vi "Data processing_average_injection (SubVI).vi"(0 "Measurement input":string) -> (20 "output cluster 2":T1, 27 "output cluster":cluster{bool, bool, bool, bool, bool, bool})   [LabVIEW 2014]
uses:
  <vilib>/Analysis/NI_AALBase.lvlib
  <vilib>/Analysis/baseanly.llb/Mean (DBL).vi
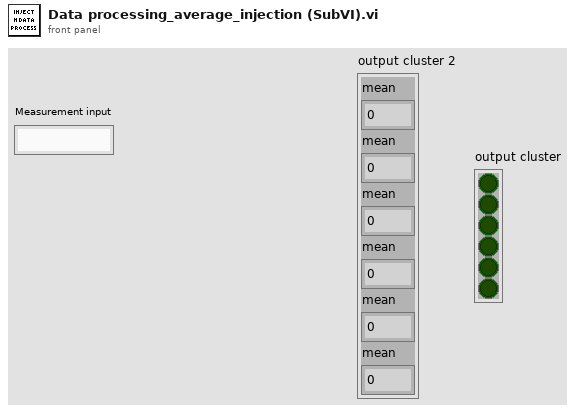
[diagram p1: front panel]
types:
  T1 = cluster{"mean":dbl, "mean":dbl, "mean":dbl, "mean":dbl, "mean":dbl, "mean":dbl}
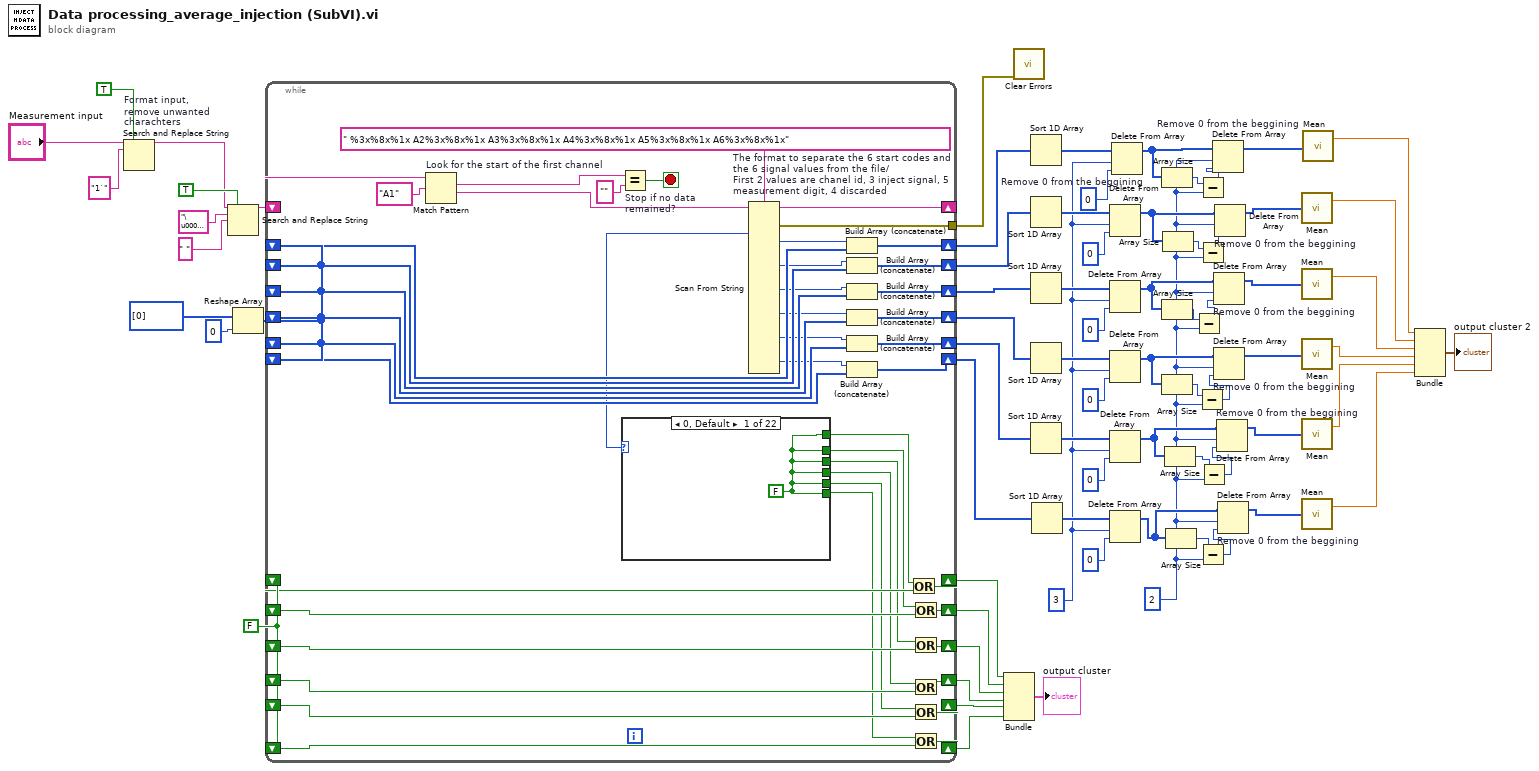
[diagram p0: block diagram]
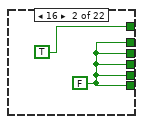
[diagram p2: hidden frame]
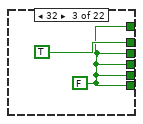
[diagram p3: hidden frame]
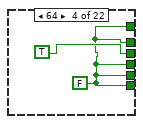
[diagram p4: hidden frame]
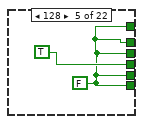
[diagram p5: hidden frame]
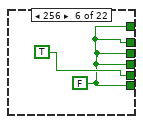
[diagram p6: hidden frame]
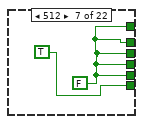
[diagram p7: hidden frame]
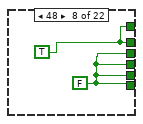
[diagram p8: hidden frame]
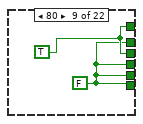
[diagram p9: hidden frame]
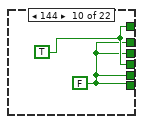
[diagram p10: hidden frame]
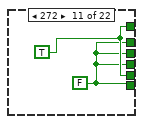
[diagram p11: hidden frame]
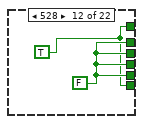
[diagram p12: hidden frame]
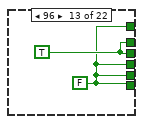
[diagram p13: hidden frame]
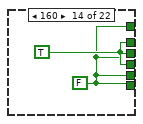
[diagram p14: hidden frame]
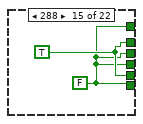
[diagram p15: hidden frame]
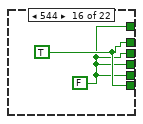
[diagram p16: hidden frame]
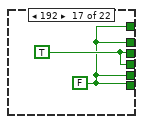
[diagram p17: hidden frame]
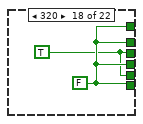
[diagram p18: hidden frame]
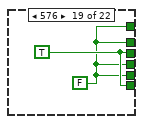
[diagram p19: hidden frame]
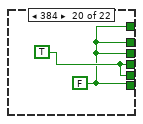
[diagram p20: hidden frame]
diagram:
  w30 = 3
  w1 = 2
  w53 = FALSE
  n1 = Search and Replace String "Format input, \nremove unwanted charachters"(replace all?=TRUE ("replace all? (F)"), input string="Measurement input", search string="1`") -> (result string=w63:string)  [unwired: 5 in, 3 out]
  n2 = Search and Replace String(replace all?=TRUE ("replace all? (F)"), input string=w63, search string="\u0003\u0002", replace string=" " ("replace string (\"\")")) -> (result string=w66:string)  [unwired: 4 in, 3 out]
  n3 = Reshape Array(i32[] [0], 0 ("dimension size")) -> (w70:i32[])
  n4 = while {
    shift-right: [w110] -> _
    shift-left: w66 -> [w114]
    tunnel: [w109] -> w68
    shift-right: [w108] -> w41
    shift-left: w70 -> [w102]
    shift-right: [w107] -> w40
    shift-left: w70 -> [w101]
    shift-right: [w106] -> w38
    shift-left: w70 -> [w100]
    shift-right: [w105] -> w36
    shift-left: w70 -> [w99]
    shift-right: [w104] -> w34
    shift-left: w70 -> [w98]
    shift-right: [w103] -> w32
    shift-left: w70 -> [w97]
    shift-right: [w90] -> w24
    shift-left: w53 -> [w89]
    shift-right: [w88] -> w25
    shift-left: w53 -> [w83]
    shift-right: [w87] -> w26
    shift-left: w53 -> [w82]
    shift-right: [w86] -> w27
    shift-left: w53 -> [w81]
    shift-right: [w85] -> w28
    shift-left: w53 -> [w80]
    shift-right: [w84] -> w29
    shift-left: w53 -> [w79]
    stop <- w111 stop-if-true
    w117 = " %3x%8x%1x A2%3x%8x%1x A3%3x%8x%1x A4%3x%8x%1x A5%3x%8x%1x A6%3x%8x%1x"  # The format to separate the 6 start codes and the 6 signal values from the file/  First 2 values are chanel id, 3 inject signal, 5 measurement digit, 4 discarded
    n5 = Match Pattern "Look for the start of the first channel"(string=w114, regular expression="A1") -> (match substring=w113:string, after substring=w115:string)  [unwired: 1 in, 2 out]
    n6 = Equal? "Stop if no data remained?"(x=w113, y="") -> (x = y?=w111:bool)
    n7 = Scan From String(format string=w117, input string=w115) -> (remaining string=w110:string, error out=w109:errorcluster, output 1=w78:u32, output 2=w96:u32, output 5=w95:u32, output 8=w94:u32, output 11=w93:u32, output 14=w92:u32, output 17=w91:u32)  [unwired: 31 in, 1 out]
    n8 = case shown="0, Default" w78 {
      tunnel: [w118 TRUE w121 w123 w125 w127 w129 w131 w134 w136 w138 w139 w141 w143 w145 w147 w149 w152 w153 w155 w157 w160] -> w77
      tunnel: [w118 w120 TRUE w123 w125 w127 w129 w131 w133 w135 w137 w140 w142 w144 w146 w148 w149 w152 w153 w155 w157 w160] -> w76
      tunnel: [w118 w120 w121 TRUE w125 w127 w129 w132 w134 w135 w137 w140 w142 w143 w145 w147 w150 w151 w154 w155 w157 w160] -> w75
      tunnel: [w118 w120 w121 w123 TRUE w127 w129 w132 w133 w136 w137 w140 w141 w144 w145 w147 w150 w152 w153 w156 w158 w160] -> w74
      tunnel: [w118 w120 w121 w123 w125 TRUE w129 w132 w133 w135 w138 w140 w141 w143 w146 w147 w149 w151 w153 w156 w157 w159] -> w73
      tunnel: [w118 w120 w121 w123 w125 w127 TRUE w132 w133 w135 w137 w139 w141 w143 w145 w148 w149 w152 w154 w155 w158 w159] -> w72
      frame 0, Default {
        w118 = FALSE
      }
      frame 16 {
        w120 = FALSE
      }
      frame 32 {
        w121 = FALSE
      }
      frame 64 {
        w123 = FALSE
      }
      frame 128 {
        w125 = FALSE
      }
      frame 256 {
        w127 = FALSE
      }
      frame 512 {
        w129 = FALSE
      }
      frame 48 {
        w131 = TRUE
        w132 = FALSE
      }
      frame 80 {
        w134 = TRUE
        w133 = FALSE
      }
      frame 144 {
        w136 = TRUE
        w135 = FALSE
      }
      frame 272 {
        w138 = TRUE
        w137 = FALSE
      }
      frame 528 {
        w139 = TRUE
        w140 = FALSE
      }
      frame 96 {
        w142 = TRUE
        w141 = FALSE
      }
      frame 160 {
        w144 = TRUE
        w143 = FALSE
      }
      frame 288 {
        w146 = TRUE
        w145 = FALSE
      }
      frame 544 {
        w148 = TRUE
        w147 = FALSE
      }
      frame 192 {
        w150 = TRUE
        w149 = FALSE
      }
      frame 320 {
        w151 = TRUE
        w152 = FALSE
      }
      frame 576 {
        w154 = TRUE
        w153 = FALSE
      }
      frame 384 {
        w156 = TRUE
        w155 = FALSE
      }
      frame 640 {
        w158 = TRUE
        w157 = FALSE
      }
      frame 768 {
        w159 = TRUE
        w160 = FALSE
      }
    }
    n9 = Build Array (concatenate)(w96, w102) -> (w108:u32[])
    n10 = Build Array (concatenate)(w95, w101) -> (w107:u32[])
    n11 = Build Array (concatenate)(w94, w100) -> (w106:u32[])
    n12 = Build Array (concatenate)(w93, w99) -> (w105:u32[])
    n13 = Build Array (concatenate)(w92, w98) -> (w104:u32[])
    n14 = Build Array (concatenate)(w91, w97) -> (w103:u32[])
    n15 = Or(x=w77, y=w89) -> (x .or. y?=w90:bool)
    n16 = Or(x=w76, y=w83) -> (x .or. y?=w88:bool)
    n17 = Or(x=w75, y=w82) -> (x .or. y?=w87:bool)
    n18 = Or(x=w74, y=w81) -> (x .or. y?=w86:bool)
    n19 = Or(x=w73, y=w80) -> (x .or. y?=w85:bool)
    n20 = Or(x=w72, y=w79) -> (x .or. y?=w84:bool)
  }
  n21 = Bundle(w24, w25, w26, w27, w28, w29) -> (→"output cluster":cluster{bool, bool, bool, bool, bool, bool})  [unwired: 1 in]
  n22 = call <vilib>:"Clear Errors.vi"("error in (no error)"=w68) -> ()  [unwired: 5 in, 2 out]
  n23 = Sort 1D Array(array=w41) -> (sorted array=w14:u32[])
  n24 = Sort 1D Array(array=w40) -> (sorted array=w39:u32[])
  n25 = Sort 1D Array(array=w38) -> (sorted array=w37:u32[])
  n26 = Sort 1D Array(array=w36) -> (sorted array=w35:u32[])
  n27 = Sort 1D Array(array=w34) -> (sorted array=w33:u32[])
  n28 = Sort 1D Array(array=w32) -> (sorted array=w31:u32[])
  n29 = Delete From Array(array=w39, length=w30, index=0) -> (array with subset deleted=w46:u32[])  [unwired: 1 out]
  n30 = Delete From Array(array=w37, length=w30, index=0) -> (array with subset deleted=w47:u32[])  [unwired: 1 out]
  n31 = Delete From Array(array=w35, length=w30, index=0) -> (array with subset deleted=w48:u32[])  [unwired: 1 out]
  n32 = Delete From Array(array=w33, length=w30, index=0) -> (array with subset deleted=w49:u32[])  [unwired: 1 out]
  n33 = Delete From Array(array=w31, length=w30, index=0) -> (array with subset deleted=w50:u32[])  [unwired: 1 out]
  n34 = Delete From Array "Remove 0 from the beggining"(array=w14, length=w30, index=0) -> (array with subset deleted=w52:u32[])  [unwired: 1 out]
  n35 = Array Size(array=w52) -> (size(s)=w12:i32)
  n36 = Array Size(array=w47) -> (size(s)=w8:i32)
  n37 = Array Size(array=w48) -> (size(s)=w6:i32)
  n38 = Array Size(array=w46) -> (size(s)=w11:i32)
  n39 = Array Size(array=w49) -> (size(s)=w4:i32)
  n40 = Array Size(array=w50) -> (size(s)=w2:i32)
  n41 = Subtract(x=w8, y=w1) -> (x-y=w9:i32)
  n42 = Subtract(x=w6, y=w1) -> (x-y=w7:i32)
  n43 = Subtract(x=w12, y=w1) -> (x-y=w13:i32)
  n44 = Subtract(x=w11, y=w1) -> (x-y=w10:i32)
  n45 = Subtract(x=w2, y=w1) -> (x-y=w3:i32)
  n46 = Subtract(x=w4, y=w1) -> (x-y=w5:i32)
  n47 = Delete From Array "Remove 0 from the beggining"(array=w52, length=w1, index=w13) -> (array with subset deleted=w15:u32[])  [unwired: 1 out]
  n48 = Delete From Array "Remove 0 from the beggining"(array=w47, length=w1, index=w9) -> (array with subset deleted=w44:u32[])  [unwired: 1 out]
  n49 = Delete From Array "Remove 0 from the beggining"(array=w48, length=w1, index=w7) -> (array with subset deleted=w43:u32[])  [unwired: 1 out]
  n50 = Delete From Array "Remove 0 from the beggining"(array=w46, length=w1, index=w10) -> (array with subset deleted=w45:u32[])  [unwired: 1 out]
  n51 = Delete From Array "Remove 0 from the beggining"(array=w49, length=w1, index=w5) -> (array with subset deleted=w42:u32[])  [unwired: 1 out]
  n52 = Delete From Array "Remove 0 from the beggining"(array=w50, length=w1, index=w3) -> (array with subset deleted=w51:u32[])  [unwired: 1 out]
  n53 = call-poly <vilib>:"Mean.vi"("X"=w45) -> ("mean"=w18:dbl)  [unwired: 1 out]
  n54 = call-poly <vilib>:"Mean.vi"("X"=w44) -> ("mean"=w19:dbl)  [unwired: 1 out]
  n55 = call-poly <vilib>:"Mean.vi"("X"=w43) -> ("mean"=w22:dbl)  [unwired: 1 out]
  n56 = call-poly <vilib>:"Mean.vi"("X"=w42) -> ("mean"=w21:dbl)  [unwired: 1 out]
  n57 = call-poly <vilib>:"Mean.vi"("X"=w51) -> ("mean"=w20:dbl)  [unwired: 1 out]
  n58 = call-poly <vilib>:"Mean.vi"("X"=w15) -> ("mean"=w16:dbl)  [unwired: 1 out]
  n59 = Bundle("mean"=w16, "mean"=w18, "mean"=w19, "mean"=w22, "mean"=w21, "mean"=w20) -> (→"output cluster 2":T1)  [unwired: 1 in]
